vi "Arduino Writer.vi"   [LabVIEW 2014]
uses:
  Support Code/Robot Global Data.vi
panel:
  # "Remember: STOP before unplugging\nARDUINO!!!!!"
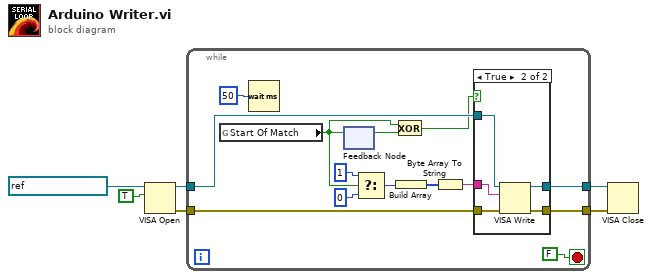
[diagram p0: block diagram]
diagram:
  n1 = VISA Open(duplicate session (F)=TRUE, VISA resource name=refnum<visa-resource-name> "ASRL3::INSTR") -> (VISA resource name=w3:refnum<visa-resource-name>, error out=w2:errorcluster)  [unwired: 1 in, 2 out]
  n2 = while {
    tunnel: w3 -> [w20]
    tunnel: [w18] -> w6
    tunnel: w2 -> [w16]
    tunnel: [w15] -> w5
    stop <- FALSE stop-if-true
    n3 = global read "Robot Global Data.vi" "Start Of Match"() -> (w7:bool)
    n4 = Wait (ms)(milliseconds to wait=u32 50) -> ()  [unwired: 1 out]
    n5 = feedback #1() -> (w8:bool)  [unwired: 1 in]
    n6 = feedback-in #1(w7) -> ()
    n7 = Select(t=u8 1 ("element"), s=w7, f=u8 0) -> (s? t:f=w14:u8)
    n8 = Exclusive Or(1:w8, 2:w7) -> (0:w9:bool)
    n9 = Build Array(w14) -> (w11:u8[])
    n10 = Byte Array To String(unsigned byte array=w11) -> (string=w19:string)
    n11 = case shown="True" w9 {
      tunnel: w20 -> [w22 w27]
      tunnel: w19 -> [_ w26]
      tunnel: [w22 w25] -> w18
      tunnel: w16 -> [w21 w24]
      tunnel: [w21 w23] -> w15
      frame False {
      }
      frame True {
        n12 = VISA Write(VISA resource name=w27, write buffer=w26, error in (no error)=w24) -> (VISA resource name out=w25:refnum<visa-resource-name>, error out=w23:errorcluster)  [unwired: 1 out]
      }
    }
  }
  n13 = VISA Close(VISA resource name=w6, error in (no error)=w5) -> ()  [unwired: 1 out]
